vi "Spartan HTTP Receive Command.vi"(4 "error in (no error)":errorcluster, 7 "HTTP Data":T4 {"object data"."time" format="%0.2f"}) -> (0 "error out":errorcluster, 2 "request info":T3={"process"=FALSE, "accessed document"="", "request type"=enum."CGI Movie", "reply"={"content"="", "header"="", "keep alive"=FALSE, "don't write"=FALSE}, "script alias"=FALSE}, 3 "HTTP Data 2":T4 {"object data"."time" format="%0.2f"})   [LabVIEW 2011]
uses:
  Spartan HTTP Session.ctl
  ITK EXT/http/http_obj.llb/HTTP Session Data.ctl
  ITK EXT/utils/keyedarr.llb/Keyed Array.ctl
  ITK EXT/http/http1.llb/HTTP Request Type.ctl
  ITK EXT/http/cgi.llb/CGI Reply.ctl
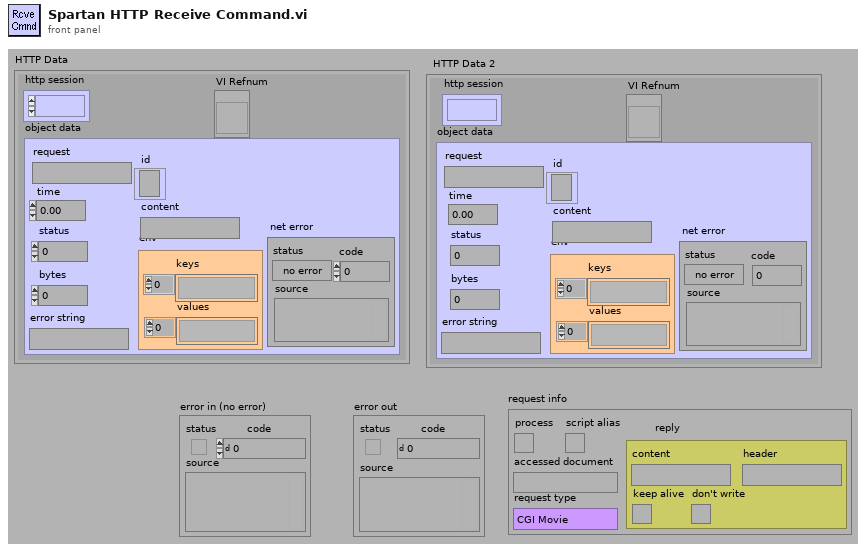
[diagram p1: front panel]
types:
  T1 = typedef "HTTP Request Type.ctl" = enum16{"Default", "Panel Picture", "Panel Movie", "CGI Movie"}
  T2 = typedef "CGI Reply.ctl" = cluster{"content":string, "header":string, "keep alive":bool, "don't write":bool}
  T3 = cluster{"process":bool, "accessed document":string, "request type":T1, "reply":T2, "script alias":bool}
  T4 = typedef "Spartan HTTP Session.ctl" = cluster{"http session":refnum<k1>, "object data":T5, "VI Refnum":refnum<vi>}
  T5 = typedef "HTTP Session Data.ctl" = cluster{"request":string, "time":dbl, "status":i32, "error string":string, "bytes":i32, "env":T6, "content":string, "id":refnum<k5>, "net error":errorcluster}
  T6 = typedef "Keyed Array.ctl" = cluster{"keys":string[], "values":string[]}
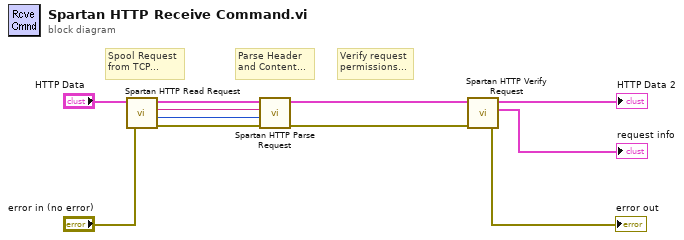
[diagram p0: block diagram]
diagram:
  # "Verify request\npermissions..."
  # "Parse Header\nand Content..."
  # "Spool Request\nfrom TCP..."
  n1 = call "Spartan HTTP Read Request.vi"("error in (no error)"="error in (no error)", "HTTP Session (empty)"="HTTP Data") -> ("error out"=w11:errorcluster, "Content Length"=w8:i32, "HTTP Request"=w1:string, "dup http session"=w10:T4)  [unwired: 2 out]
  n2 = call "Spartan HTTP Parse Request.vi"("error in (no error)"=w11, "Content-length (-1)"=w8, "HTTP Request (\"\")"=w1, "HTTP Data"=w10) -> ("error out"=w3:errorcluster, "dup http session"=w7:T4)  [unwired: 1 in, 5 out]
  n3 = call "Spartan HTTP Verify Request.vi"("error in (no error)"=w3, "HTTP Data"=w7) -> ("error out"=→"error out":errorcluster, "request info"=→"request info":T3, "dup http session"=→"HTTP Data 2":T4)  [unwired: 3 out]
